vi "check_dll_cpu_use.vi"() -> ()   [LabVIEW 2020]
panel:
  in  "position_llh":string="36.318462,138.996902,100"
  in  "update":bool
  in  "Run dll":bool
  in  "Sample rate":dbl=200000.0
  in  "Time Cycle":u32=100
  in  "dll Path":path=path "C:/Users/duyga/OneDrive/デスクトップ/WORKS/Nissan GPS/build dll/GPS_SIM_GENERATE_IQ_v2.dll"
  in  "Rinex file":path=path "C:/Users/duyga/OneDrive/デスクトップ/WORKS/Nissan GPS/build dll/brdc0010.22n"
  out "Numeric":i32
  in  "stop":bool
  out "output":i16[](array[numeric])
  out "error out":errorcluster
  in  "param(llh)":string="-l 36.318462,138.996902,100"
  # "iq8_buff[isamp] = iq_buff[isamp]>>4;"
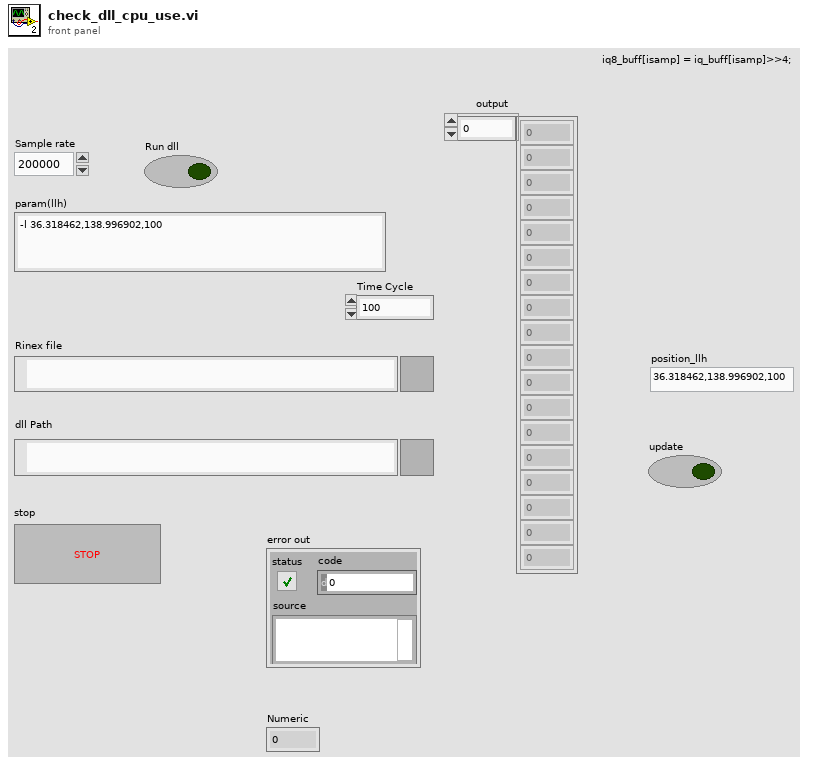
[diagram p1: front panel]
types:
  T1 = enum16{"read_RINEX", "settings", "generate_100ms"}
  T2 = enum16{"read_RINEX", "settings", "generate_100ms", "update_position"}
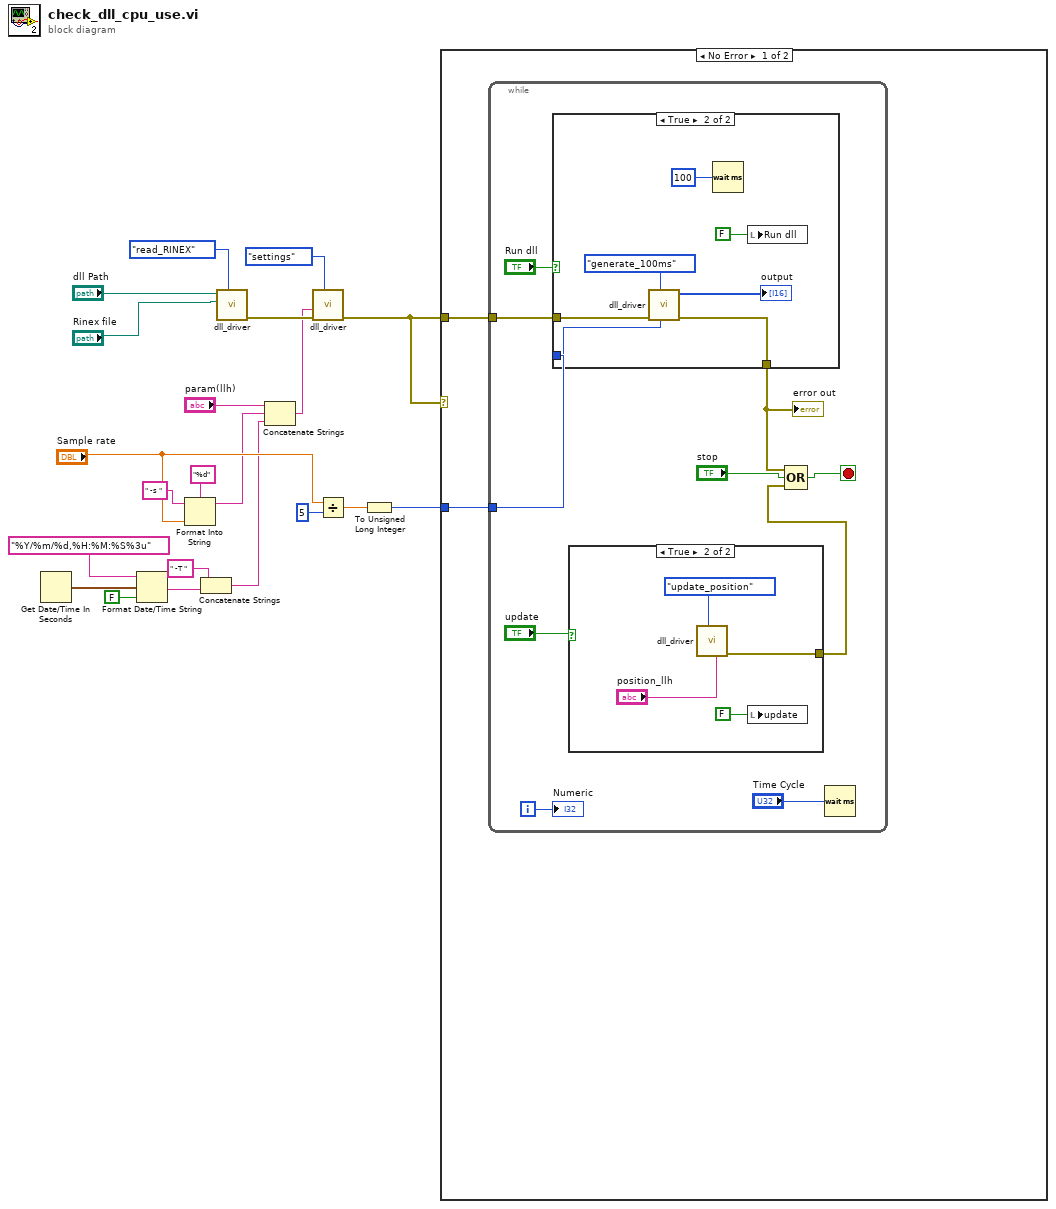
[diagram p0: block diagram]
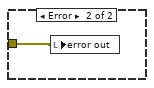
[diagram p4: hidden frame]
diagram:
  n1 = Get Date/Time In Seconds() -> (seconds since 1Jan1904=w20:timestamp)
  n2 = Format Date/Time String(time format string (%c)="%Y/%m/%d,%H:%M:%S%3u", seconds (now)=w20, UTC format=FALSE) -> (date/time string=w21:string)
  n3 = Format Into String(format string="%d", initial string=" -s ", "Sample rate") -> (resulting string=w2:string)  [unwired: 1 in, 1 out]
  n4 = Concatenate Strings(" -T " ("string"), w21) -> (w1:string)
  n5 = call "dll_driver.vi"("dll state"=T1."read_RINEX", "Rinex file"="Rinex file", "dll Path"="dll Path") -> ("error out"=w12:errorcluster)  [unwired: 7 in, 1 out]
  n6 = Concatenate Strings("param(llh)", w2, w1) -> (w10:string)
  n7 = call "dll_driver.vi"("dll state"=T1."settings", "error in"=w12, "params"=w10) -> ("error out"=w9:errorcluster)  [unwired: 7 in, 1 out]
  n8 = Divide(x="Sample rate", y=5) -> (x/y=w7:dbl)
  n9 = To Unsigned Long Integer(number=w7) -> (unsigned 32bit integer=w6:u32)
  n10 = case shown="No Error" w9 {
    tunnel: w9 -> [w23 w46]
    tunnel: w6 -> [w22 _]
    frame No Error {
      n11 = while {
        tunnel: w23 -> [w31]
        tunnel: w22 -> [w30]
        i -> [w33]
        stop <- w24 stop-if-true
        n12 = case shown="True" "Run dll" {
          tunnel: w31 -> [w38 w45]
          tunnel: [w38 w42] -> w26
          tunnel: w30 -> [_ w41]
          frame False {
          }
          frame True {
            n13 = call "dll_driver.vi"("buffer size"=w41, "dll state"=T1."generate_100ms", "error in"=w45) -> ("error out"=w42:errorcluster, "output"=→"output":i16[])  [unwired: 7 in]
            n14 = Wait (ms)(milliseconds to wait=u32 100) -> ()  [unwired: 1 out]
            n15 = local write "Run dll"(FALSE ("Run dll")) -> ()
          }
        }
        "error out" <- w26
        n16 = case shown="True" "update" {
          tunnel: [_ w35] -> w25
          frame False {
          }
          frame True {
            n17 = call "dll_driver.vi"("position_llh"="position_llh", "dll state"=T2."update_position") -> ("error out"=w35:errorcluster)  [unwired: 8 in, 1 out]
            n18 = local write "update"(FALSE ("update")) -> ()
          }
        }
        n19 = Compound Arithmetic op=OR(w26, "stop", w25) -> (w24:bool)
        n20 = Wait (ms)(milliseconds to wait="Time Cycle") -> ()  [unwired: 1 out]
        "Numeric" <- w33
      }
    }
    frame Error {
      n21 = local write "error out"(w46) -> ()
    }
  }
